vi "dfd_nMAC_CircSubN(nCh).vi"(4 "bufSize*#ch":fxp<+,16,16>, 6 "curChIdx":fxp<+,16,16>, 10 "#ch":fxp<+,16,16>, 11 "idxIn":fxp<+,16,16>) -> (3 "idxOut":fxp<+,16,16>)   [LabVIEW 2017]
uses:
  <vilib>/rvi/FXPMathLib/basic elements/FxpAddSub/XNode/nifxpmath_AddSub.xnode
  <vilib>/rvi/FXPMathLib/sim/FxpSim.dll
panel:
  in  "Enable":bool
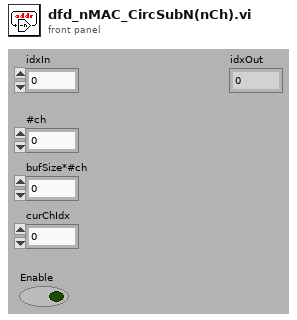
[diagram p1: front panel]
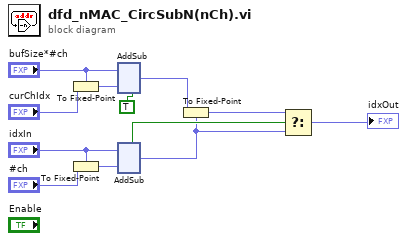
[diagram p0: block diagram]
diagram:
  n1 = To Fixed-Point(fixed-point type="bufSize*#ch", number="curChIdx") -> (fixed-point=w8:fxp<+,16,16>)
  n2 = To Fixed-Point(fixed-point type="idxIn", number="#ch") -> (fixed-point=w6:fxp<+,16,16>)
  n3 = xnode "AddSub"("x"="bufSize*#ch", "y"=w8, "borrow-in"=TRUE) -> ("s"=w10:fxp<+,16,16>)  [unwired: 1 out]
  n4 = xnode "AddSub"("x"="idxIn", "y"=w6) -> ("s"=w1:fxp<+,16,16>, "borrow-out"=w11:bool)
  n5 = To Fixed-Point(fixed-point type=w1, number=w10) -> (fixed-point=w2:fxp<+,16,16>)
  n6 = Select(t=w2, s=w11, f=w1) -> (s? t:f=→"idxOut":fxp<+,16,16>)
